vi "UI_ctrl_fgv2.vi"(7 "cmd":enum16{"read", "create"}(ring), 11 "UI in":T1) -> (3 "UI out":T1)   [LabVIEW 2016]
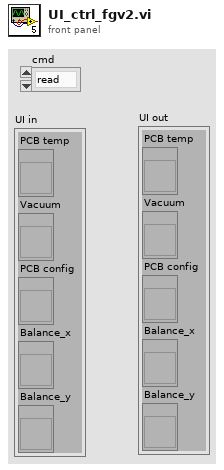
[diagram p1: front panel]
types:
  T1 = cluster{"PCB temp":refnum<vi>, "Vacuum":refnum<vi>, "PCB config":refnum<vi>, "Balance_x":refnum<vi>, "Balance_y":refnum<vi>}
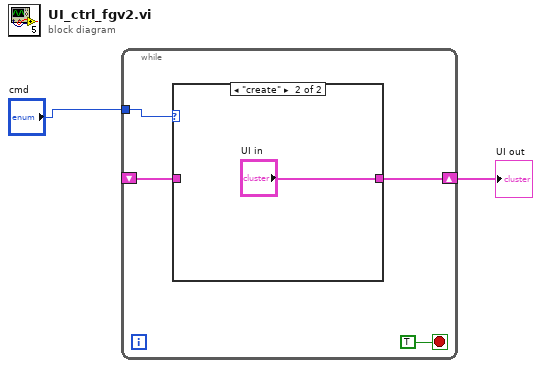
[diagram p0: block diagram]
diagram:
  n1 = while {
    tunnel: "cmd" -> [w6]
    shift-right: [w4] -> w1
    shift-left: _ -> [w3]
    stop <- TRUE stop-if-true
    n2 = case shown="\"create\"" w6 {
      tunnel: [w7 "UI in"] -> w4
      tunnel: w3 -> [w7 _]
      frame "read", Default {
      }
      frame "create" {
      }
    }
  }
  "UI out" <- w1
